vi "TempMain.vi"() -> ()   [LabVIEW 2016]
uses:
  <vilib>/FPGAPlugInAG/cRIO-9039 (Sync)/niLvFpga_Open_cRIO-9039 (Sync).vi
  <vilib>/rvi/interface/common/dynamic/niFpgaDynamicAddResources.vi
  <vilib>/FPGAPlugInAG/Dynamic/niLvFpga_Abort_Dynamic.vi
  <vilib>/FPGAPlugInAG/Dynamic/niLvFpga_Reset_Dynamic.vi
  <vilib>/FPGAPlugInAG/Dynamic/niLvFpga_Run_Dynamic.vi
  <vilib>/Utility/error.llb/Error Cluster From Error Code.vi
  <vilib>/rvi/errors/niLvFpgaAdjustHostInterfaceError.vi
  <vilib>/FPGAPlugInAG/Dynamic/niLvFpga_Close_Dynamic.vi
  <vilib>/rvi/interface/nirviOpenFPGA/nirviOpenFPGA.xnode
  FPGA Bitfiles/M1M3SupportSimulator.lvbitx
  <vilib>/rvi/interface/nirviMethod/nirviMethod.xnode
  <vilib>/rvi/interface/nirviCloseFPGA/nirviCloseFPGA.xnode
  <vilib>/FPGAPlugInAG/Dynamic/niLvFpga_WriteFifo_Dynamic.vi
  <vilib>/rvi/errors/niLvFpgaMergeErrorWithErrorCode.vi
  <vilib>/FPGAPlugInAG/Dynamic/niLvFpga_ReadFifo_Dynamic.vi
panel:
  out "Data":u32[](array[numeric])
  out "error out 3":errorcluster
  out "error out 2":errorcluster
  out "error out":errorcluster
  in  "Boolean":bool
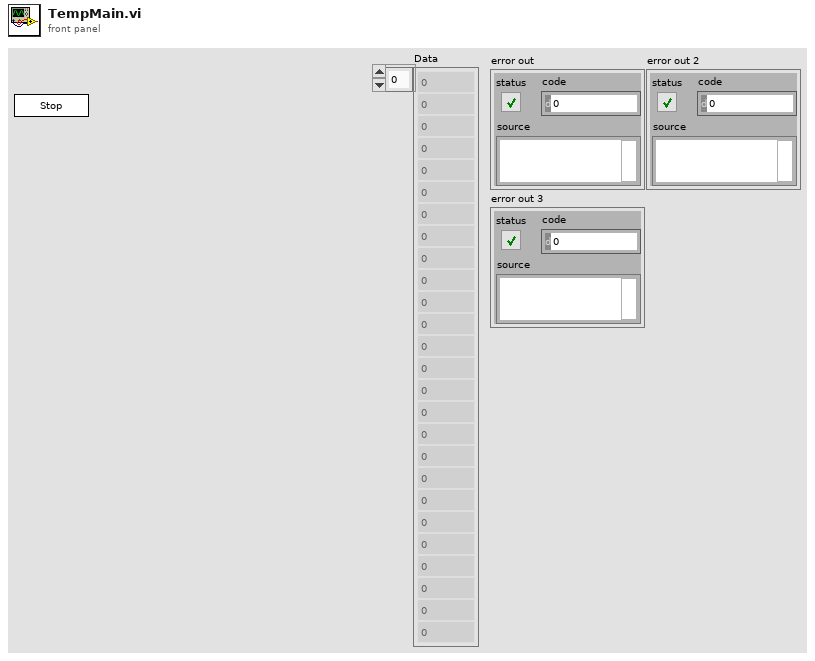
[diagram p1: front panel]
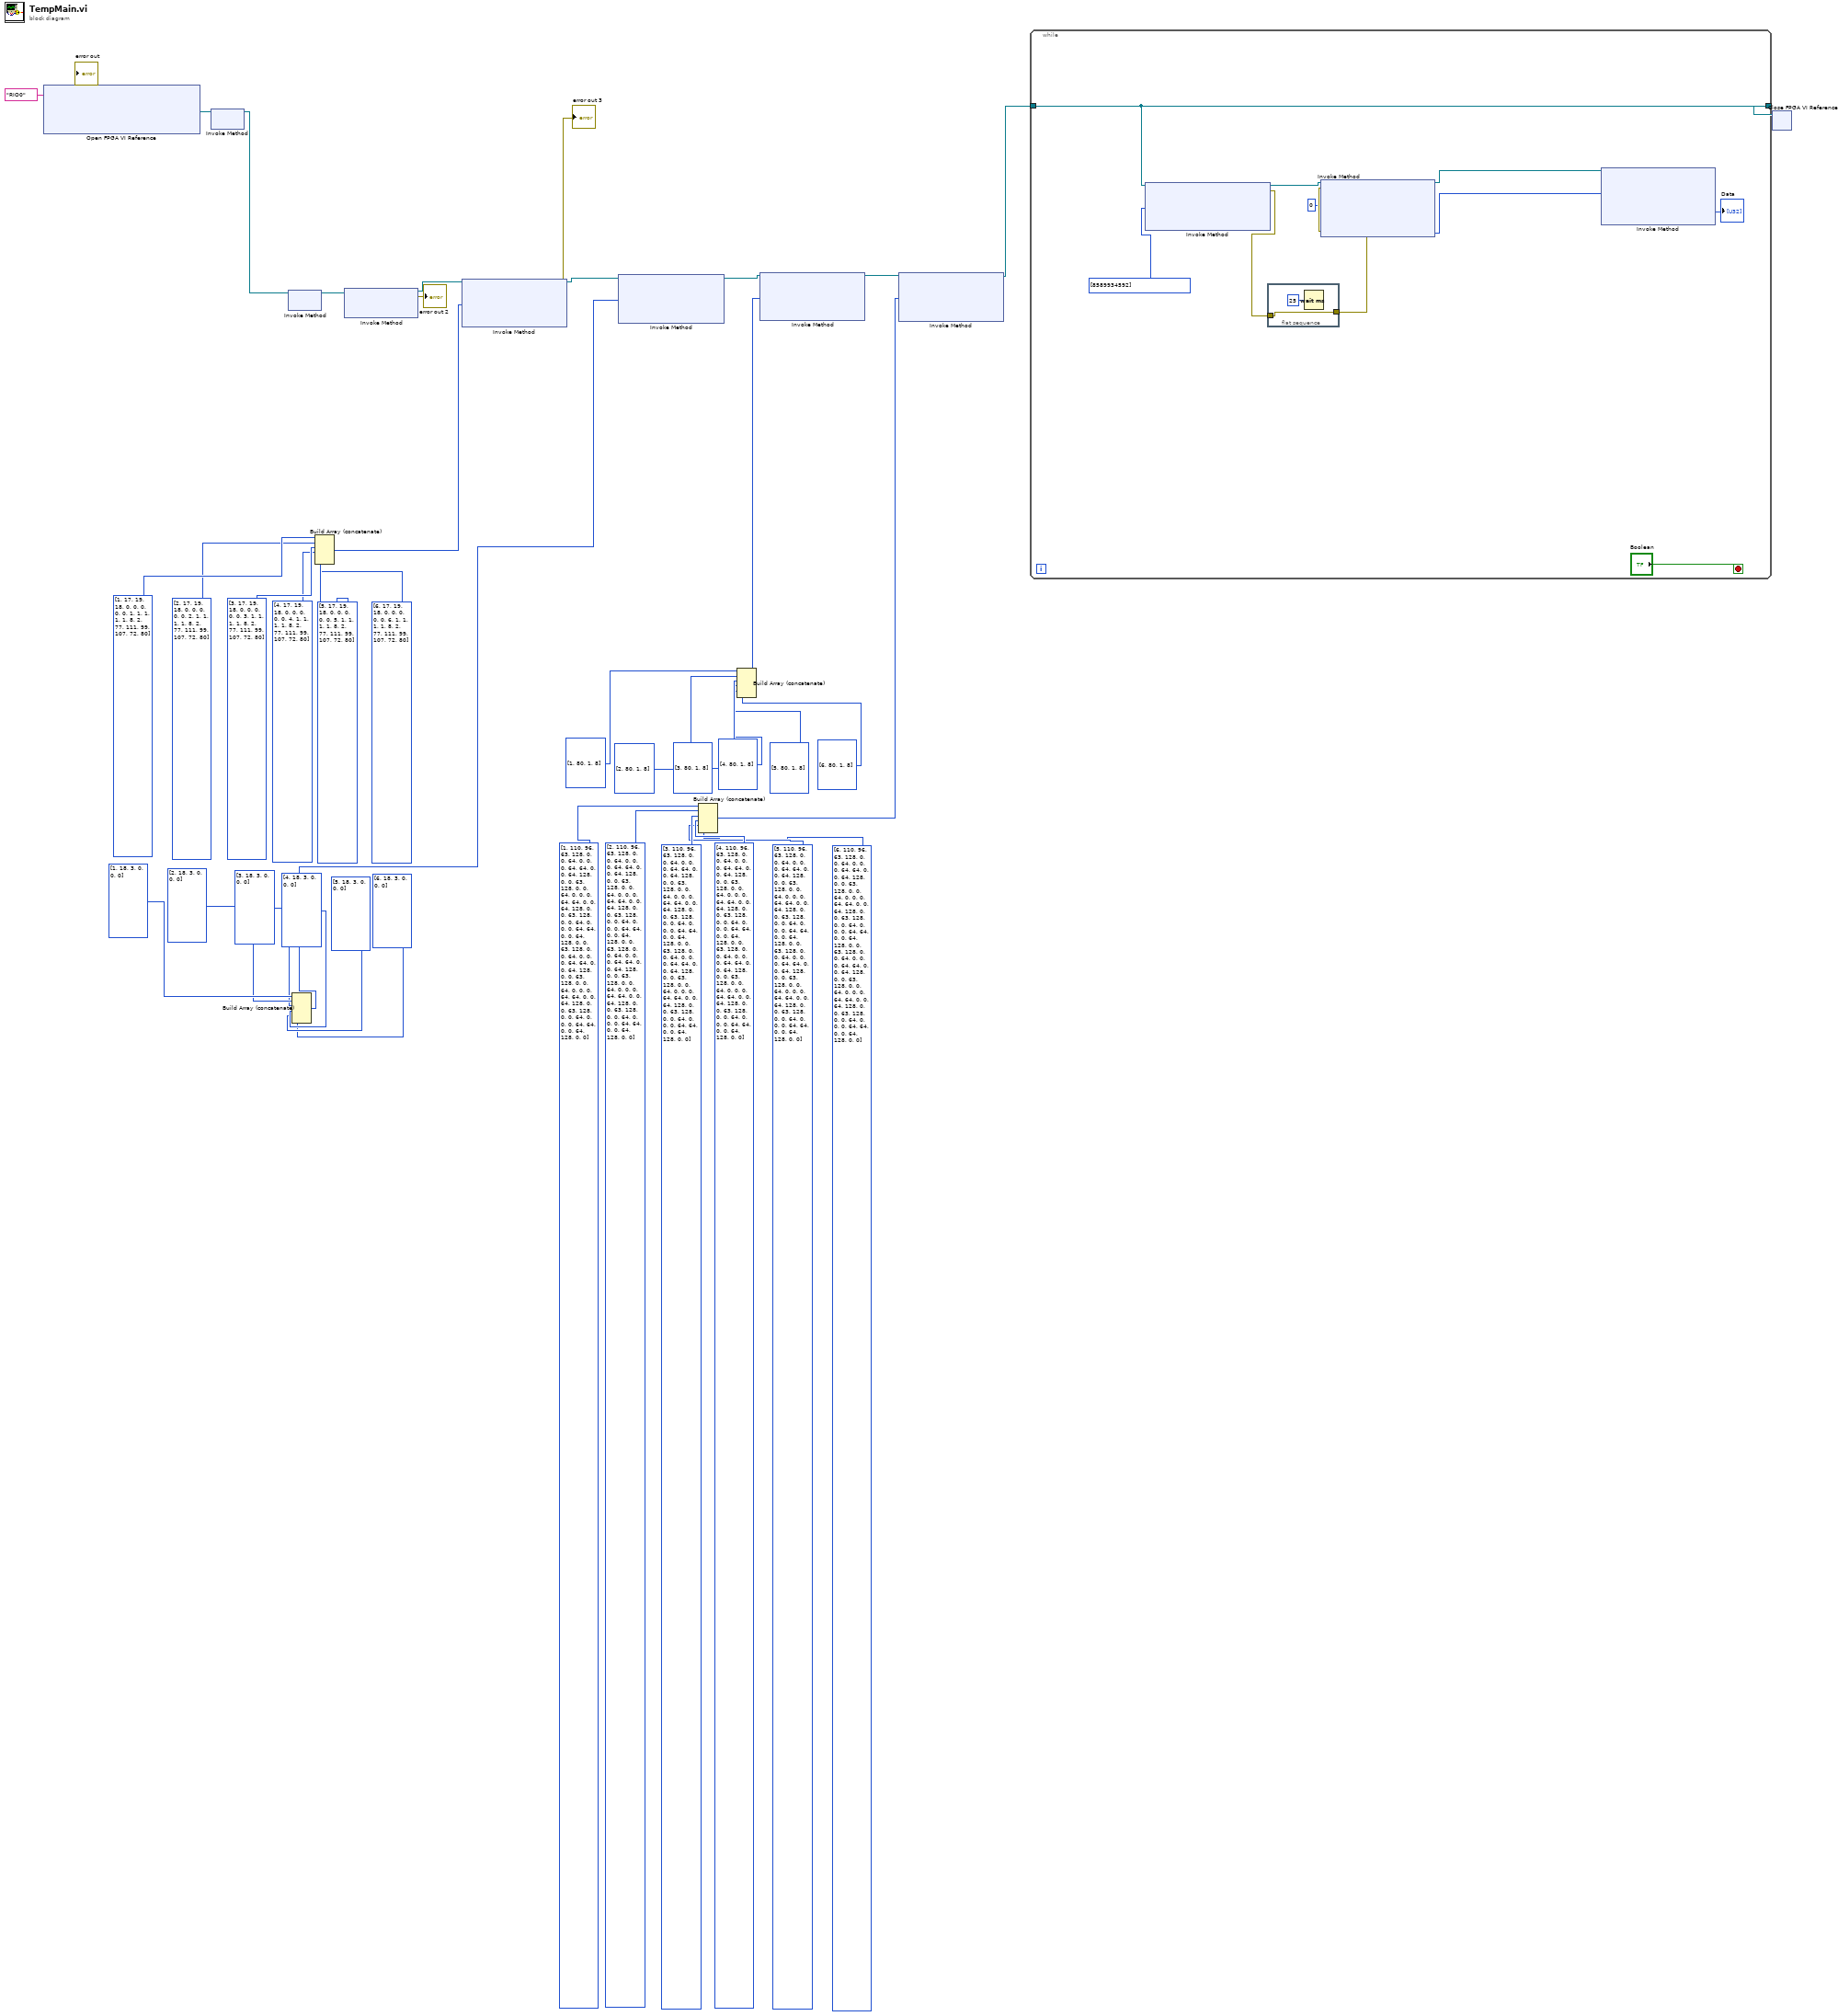
[diagram p0: block diagram]
diagram:
  n1 = xnode "Open FPGA VI Reference"("resource name"=tag "RIO0") -> ("FPGA VI Reference Out"=w41:refnum<k20>, "error out"=→"error out":errorcluster)  [unwired: 1 in]
  n2 = xnode "Invoke Method"("FPGA VI Reference In"=w41) -> ("FPGA VI Reference Out"=w40:refnum<k20>)  [unwired: 1 in, 1 out]
  n3 = xnode "Invoke Method"("FPGA VI Reference In"=w40) -> ("FPGA VI Reference Out"=w39:refnum<k20>)  [unwired: 1 in, 1 out]
  n4 = Build Array (concatenate)(u8[] [1, 18, 3, 0, 0, 0], u8[] [2, 18, 3, 0, 0, 0], u8[] [3, 18, 3, 0, 0, 0], u8[] [4, 18, 3, 0, 0, 0], u8[] [5, 18, 3, 0, 0, 0], u8[] [6, 18, 3, 0, 0, 0]) -> (w21:u8[])
  n5 = Build Array (concatenate)(u8[] [1, 17, 19, 18, 0, 0, 0, 0, 0, 1, 1, 1, 1, 1, 8, 2, 77, 111, 99, 107, 72, 80], u8[] [2, 17, 19, 18, 0, 0, 0, 0, 0, 2, 1, 1, 1, 1, 8, 2, 77, 111, 99, 107, 72, 80], u8[] [3, 17, 19, 18, 0, 0, 0, 0, 0, 3, 1, 1, 1, 1, 8, 2, 77, 111, 99, 107, 72, 80], u8[] [4, 17, 19, 18, 0, 0, 0, 0, 0, 4, 1, 1, 1, 1, 8, 2, 77, 111, 99, 107, 72, 80], u8[] [5, 17, 19, 18, 0, 0, 0, 0, 0, 5, 1, 1, 1, 1, 8, 2, 77, 111, 99, 107, 72, 80], u8[] [6, 17, 19, 18, 0, 0, 0, 0, 0, 6, 1, 1, 1, 1, 8, 2, 77, 111, 99, 107, 72, 80]) -> (w28:u8[])
  n6 = xnode "Invoke Method"("FPGA VI Reference In"=w39) -> ("FPGA VI Reference Out"=w38:refnum<k20>, "error out"=→"error out 2":errorcluster)  [unwired: 2 in]
  n7 = xnode "Invoke Method"("FPGA VI Reference In"=w38, "Data"=w28) -> ("FPGA VI Reference Out"=w37:refnum<k20>, "error out"=→"error out 3":errorcluster)  [unwired: 2 in, 1 out]
  n8 = xnode "Invoke Method"("FPGA VI Reference In"=w37, "Data"=w21) -> ("FPGA VI Reference Out"=w36:refnum<k20>)  [unwired: 2 in, 2 out]
  n9 = Build Array (concatenate)(u8[] [1, 110, 96, 63, 128, 0, 0, 64, 0, 0, 0, 64, 64, 0, 0, 64, 128, 0, 0, 63, 128, 0, 0, 64, 0, 0, 0, 64, 64, 0, 0, 64, 128, 0, 0, 63, 128, 0, 0, 64, 0, 0, 0, 64, 64, 0, 0, 64, 128, 0, 0, 63, 128, 0, 0, 64, 0, 0, 0, 64, 64, 0, 0, 64, 128, 0, 0, 63, 128, 0, 0, 64, 0, 0, 0, 64, 64, 0, 0, 64, 128, 0, 0, 63, 128, 0, 0, 64, 0, 0, 0, 64, 64, 0, 0, 64, 128, 0, 0], u8[] [2, 110, 96, 63, 128, 0, 0, 64, 0, 0, 0, 64, 64, 0, 0, 64, 128, 0, 0, 63, 128, 0, 0, 64, 0, 0, 0, 64, 64, 0, 0, 64, 128, 0, 0, 63, 128, 0, 0, 64, 0, 0, 0, 64, 64, 0, 0, 64, 128, 0, 0, 63, 128, 0, 0, 64, 0, 0, 0, 64, 64, 0, 0, 64, 128, 0, 0, 63, 128, 0, 0, 64, 0, 0, 0, 64, 64, 0, 0, 64, 128, 0, 0, 63, 128, 0, 0, 64, 0, 0, 0, 64, 64, 0, 0, 64, 128, 0, 0], u8[] [3, 110, 96, 63, 128, 0, 0, 64, 0, 0, 0, 64, 64, 0, 0, 64, 128, 0, 0, 63, 128, 0, 0, 64, 0, 0, 0, 64, 64, 0, 0, 64, 128, 0, 0, 63, 128, 0, 0, 64, 0, 0, 0, 64, 64, 0, 0, 64, 128, 0, 0, 63, 128, 0, 0, 64, 0, 0, 0, 64, 64, 0, 0, 64, 128, 0, 0, 63, 128, 0, 0, 64, 0, 0, 0, 64, 64, 0, 0, 64, 128, 0, 0, 63, 128, 0, 0, 64, 0, 0, 0, 64, 64, 0, 0, 64, 128, 0, 0], u8[] [4, 110, 96, 63, 128, 0, 0, 64, 0, 0, 0, 64, 64, 0, 0, 64, 128, 0, 0, 63, 128, 0, 0, 64, 0, 0, 0, 64, 64, 0, 0, 64, 128, 0, 0, 63, 128, 0, 0, 64, 0, 0, 0, 64, 64, 0, 0, 64, 128, 0, 0, 63, 128, 0, 0, 64, 0, 0, 0, 64, 64, 0, 0, 64, 128, 0, 0, 63, 128, 0, 0, 64, 0, 0, 0, 64, 64, 0, 0, 64, 128, 0, 0, 63, 128, 0, 0, 64, 0, 0, 0, 64, 64, 0, 0, 64, 128, 0, 0], u8[] [5, 110, 96, 63, 128, 0, 0, 64, 0, 0, 0, 64, 64, 0, 0, 64, 128, 0, 0, 63, 128, 0, 0, 64, 0, 0, 0, 64, 64, 0, 0, 64, 128, 0, 0, 63, 128, 0, 0, 64, 0, 0, 0, 64, 64, 0, 0, 64, 128, 0, 0, 63, 128, 0, 0, 64, 0, 0, 0, 64, 64, 0, 0, 64, 128, 0, 0, 63, 128, 0, 0, 64, 0, 0, 0, 64, 64, 0, 0, 64, 128, 0, 0, 63, 128, 0, 0, 64, 0, 0, 0, 64, 64, 0, 0, 64, 128, 0, 0], u8[] [6, 110, 96, 63, 128, 0, 0, 64, 0, 0, 0, 64, 64, 0, 0, 64, 128, 0, 0, 63, 128, 0, 0, 64, 0, 0, 0, 64, 64, 0, 0, 64, 128, 0, 0, 63, 128, 0, 0, 64, 0, 0, 0, 64, 64, 0, 0, 64, 128, 0, 0, 63, 128, 0, 0, 64, 0, 0, 0, 64, 64, 0, 0, 64, 128, 0, 0, 63, 128, 0, 0, 64, 0, 0, 0, 64, 64, 0, 0, 64, 128, 0, 0, 63, 128, 0, 0, 64, 0, 0, 0, 64, 64, 0, 0, 64, 128, 0, 0]) -> (w7:u8[])
  n10 = Build Array (concatenate)(u8[] [1, 80, 1, 8], u8[] [2, 80, 1, 8], u8[] [3, 80, 1, 8], u8[] [4, 80, 1, 8], u8[] [5, 80, 1, 8], u8[] [6, 80, 1, 8]) -> (w14:u8[])
  n11 = xnode "Invoke Method"("FPGA VI Reference In"=w36, "Data"=w14) -> ("FPGA VI Reference Out"=w35:refnum<k20>)  [unwired: 2 in, 2 out]
  n12 = xnode "Invoke Method"("FPGA VI Reference In"=w35, "Data"=w7) -> ("FPGA VI Reference Out"=w6:refnum<k20>)  [unwired: 2 in, 2 out]
  n13 = while {
    tunnel: w6 -> [w50]
    tunnel: [w50] -> w5
    stop <- "Boolean" stop-if-true
    n14 = xnode "Invoke Method"("FPGA VI Reference In"=w50, "Data"=u64[] [8589934592]) -> ("FPGA VI Reference Out"=w45:refnum<k20>, "error out"=w47:errorcluster)  [unwired: 2 in, 1 out]
    n15 = flat-sequence {
      tunnel: [w53] -> w48
      tunnel: w47 -> [w53]
      frame #0 {
        n16 = Wait (ms)(milliseconds to wait=u32 25) -> ()  [unwired: 1 out]
      }
    }
    n17 = xnode "Invoke Method"("FPGA VI Reference In"=w45, "error in"=w48, "Number of Elements"=u32 0) -> ("FPGA VI Reference Out"=w44:refnum<k20>, "Elements Remaining"=w43:u32)  [unwired: 1 in, 2 out]
    n18 = xnode "Invoke Method"("FPGA VI Reference In"=w44, "Number of Elements"=w43) -> ("Data"=→"Data":u32[])  [unwired: 2 in, 3 out]
  }
  n19 = xnode "Close FPGA VI Reference"("FPGA VI Reference In"=w5) -> ()  [unwired: 1 in, 1 out]
